vi "LaunchVI.vi"() -> ()   [LabVIEW 2014]
uses:
  <vilib>/ActorFramework/Actor/Actor.lvclass
  RealWorkActor/RealWorkActor/RealWorkActor.lvclass
  RealWorkActor/RealWorkActor Messages/ProgramInitial Msg/ProgramInitial Msg.lvclass
  RealWorkActor/RealWorkActor Messages/UITimeout Msg/UITimeout Msg.lvclass
  RealWorkActor/RealWorkActor Messages/Read NowTime Msg/Read NowTime Msg.lvclass
  RealWorkActor/RealWorkActor Messages/Read MsgString Msg/Read MsgString Msg.lvclass
  RealWorkActor/RealWorkActor Messages/ActionA Msg/ActionA Msg.lvclass
  RealWorkActor/RealWorkActor Messages/ActionB Msg/ActionB Msg.lvclass
  RealWorkActor/RealWorkActor Messages/ActionC Msg/ActionC Msg.lvclass
  <vilib>/ActorFramework/Stop Msg/Stop Msg.lvclass
panel:
  out "NowTime":timestamp
  out "MsgString":string
  in  "ButtonC":bool
  in  "ButtonB":bool
  in  "ButtonA":bool
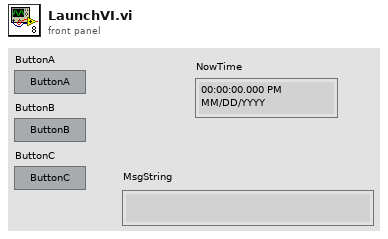
[diagram p1: front panel]
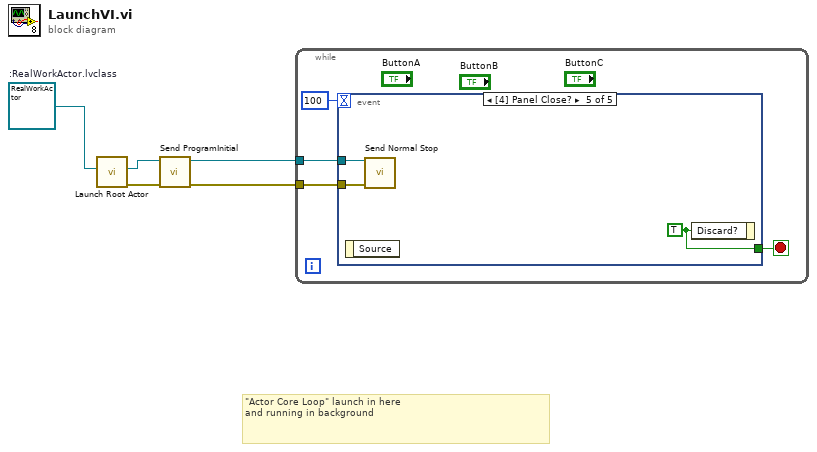
[diagram p0: block diagram]
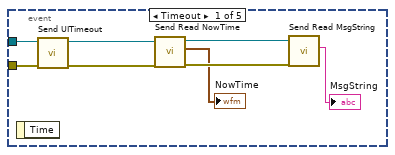
[diagram p2: hidden frame]
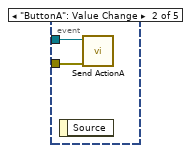
[diagram p3: hidden frame]
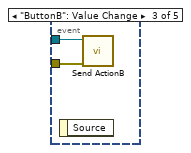
[diagram p4: hidden frame]
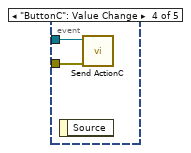
[diagram p5: hidden frame]
diagram:
  w5 = refnum<class "RealWorkActor.lvclass"> refnum  # :RealWorkActor.lvclass
  # "\"Actor Core Loop\" launch in here \nand running in background"
  n1 = call <vilib>:"Launch Root Actor.vi"("Actor"=w5) -> ("error out"=w4:errorcluster, "Actor's Enqueuer"=w2:refnum<class "Message Enqueuer.lvclass">)  [unwired: 9 in]
  n2 = call "Send ProgramInitial.vi"("error in (no error)"=w4, "Message Enqueuer"=w2) -> ("error out"=w3:errorcluster, "Message Enqueuer out"=w1:refnum<class "Message Enqueuer.lvclass">)  [unwired: 8 in]
  n3 = while {
    tunnel: w3 -> [w9]
    tunnel: w1 -> [w8]
    stop <- w6 stop-if-true
    n4 = event shown="[4] Panel Close?" {
      selector: _ -> [_ _ _ _ _]
      dyn-events: _ -> [_ _ _ _ _]
      timeout: 100 -> [_ _ _ _ _]
      tunnel: w9 -> [w17 w19 w21 w23 w25]
      tunnel: w8 -> [w16 w18 w20 w22 w24]
      tunnel: [_ _ _ _ w26] -> w6
      event Timeout {
        n5 = event-data() -> ()  [unwired: 1 in, 1 out]
        n6 = call "Send UITimeout.vi"("error in (no error)"=w17, "Message Enqueuer"=w16) -> ("error out"=w15:errorcluster, "Message Enqueuer out"=w14:refnum<class "Message Enqueuer.lvclass">)  [unwired: 8 in]
        n7 = call "Send Read NowTime.vi"("error in (no error)"=w15, "Message Enqueuer"=w14) -> ("error out"=w13:errorcluster, "NowTime"=→"NowTime":timestamp, "Message Enqueuer out"=w12:refnum<class "Message Enqueuer.lvclass">)  [unwired: 7 in]
        n8 = call "Send Read MsgString.vi"("error in (no error)"=w13, "Message Enqueuer"=w12) -> ("MsgString"=→"MsgString":string)  [unwired: 7 in, 2 out]
      }
      event "ButtonA": Value Change {
        n9 = event-data() -> ()  [unwired: 1 in, 1 out]
        n10 = call "Send ActionA.vi"("error in (no error)"=w19, "Message Enqueuer"=w18) -> ()  [unwired: 8 in, 2 out]
      }
      event "ButtonB": Value Change {
        n11 = event-data() -> ()  [unwired: 1 in, 1 out]
        n12 = call "Send ActionB.vi"("error in (no error)"=w21, "Message Enqueuer"=w20) -> ()  [unwired: 8 in, 2 out]
      }
      event "ButtonC": Value Change {
        n13 = event-data() -> ()  [unwired: 1 in, 1 out]
        n14 = call "Send ActionC.vi"("error in (no error)"=w23, "Message Enqueuer"=w22) -> ()  [unwired: 8 in, 2 out]
      }
      event Panel Close? {
        w26 = TRUE ("Discard?")
        n15 = event-data() -> ()  [unwired: 1 in, 1 out]
        n16 = call <vilib>:"Send Normal Stop.vi"("error in (no error)"=w25, "Message Enqueuer"=w24) -> ()  [unwired: 9 in, 1 out]
        n17 = event-data("Discard?"=w26) -> ()  [unwired: 1 in, 1 out]
      }
    }
  }
